vi "zero_out_masked_image_parts.vi"(10 "i32_ar_first_and_last_pixel":i32[](array[numeric]), 11 "unwrapped_Array":i16[](array[numeric])) -> (3 "Array out":i16[](array[numeric]))   [LabVIEW 2011]
doc: "Sets the values of the array that are not image pixels back to 0. This is necesseray since both the image and mask pixel were changed during the unwrapping and normalization process."
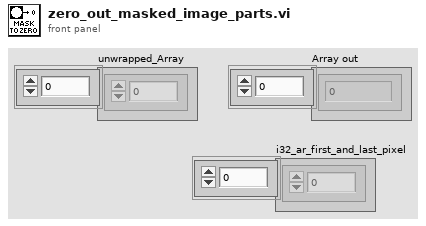
[diagram p1: front panel]
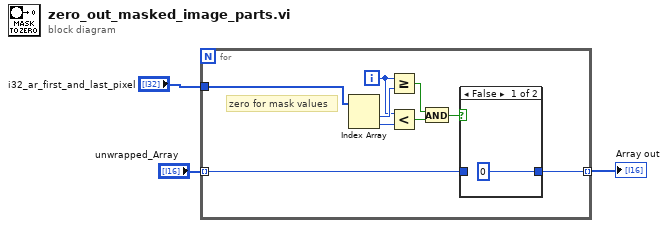
[diagram p0: block diagram]
diagram:
  n1 = for {
    tunnel: "unwrapped_Array" -> [w8] mode=indexing
    tunnel: [w9] -> w3 mode=indexing
    tunnel: "i32_ar_first_and_last_pixel" -> [w4]
    i -> [w5]
    # "zero for mask values"
    n2 = Index Array(array=w4) -> (element #1=w7:i32, element #2=w6:i32)  [unwired: 2 in]
    n3 = Greater Or Equal?(x=w5, y=w7) -> (x >= y?=w11:bool)
    n4 = Less?(x=w5, y=w6) -> (x < y?=w12:bool)
    n5 = And(x=w11, y=w12) -> (x .and. y?=w10:bool)
    n6 = case shown="False" w10 {
      tunnel: [i16 0 ("Numeric Control") w14] -> w9
      tunnel: w8 -> [_ w14]
      frame False {
      }
      frame True {
      }
    }
  }
  "Array out" <- w3
